vi "GetKey.vi"(10 "node ref in":refnum<data-value>, 11 "RVCLibrary_Bug2 in":refnum<class "RVCLibrary_Bug2.lvclass">) -> (1 "key out":cluster{"(g or v) + h":dbl, "g or v":dbl}, 2 "node ref out":refnum<data-value>, 3 "RVCLibrary_Bug2 out":refnum<class "RVCLibrary_Bug2.lvclass">)   [LabVIEW 2013, in "RVCLibrary_Bug2.lvclass"]
uses:
  RVCLibrary_Bug2.lvclass
  <vilib>/robotics/Navigation/shared/MapNode/AbstractDstarNode/NI_Robotics_AbstractDstarNode.lvclass
  RVCLibrary_Bug2.lvclass/RVCLibrary_Bug2.ctl
panel:
  in  "epsilon current":dbl
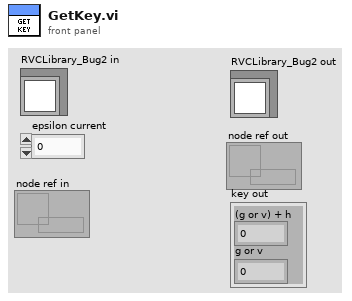
[diagram p1: front panel]
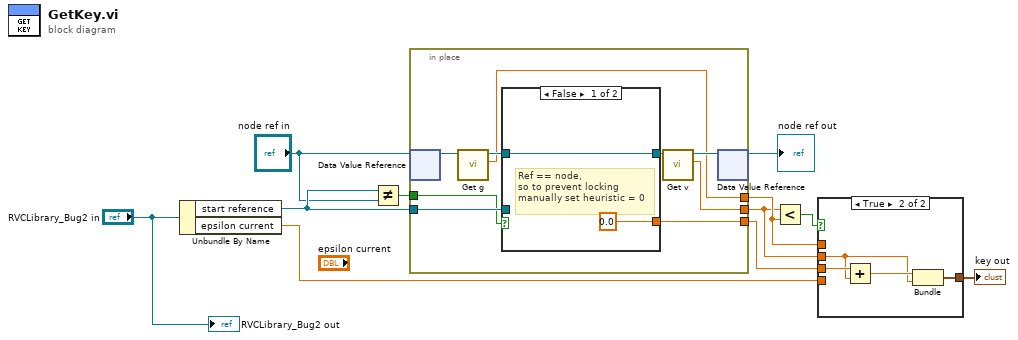
[diagram p0: block diagram]
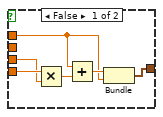
[diagram p2: hidden frame]
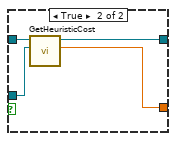
[diagram p3: hidden frame]
diagram:
  n1 = Unbundle By Name("RVCLibrary_Bug2 in") -> ("start reference"=w3:refnum<data-value>, "epsilon current"=w5:dbl)
  n2 = Not Equal?(x=w3, y="node ref in") -> (x != y?=w4:bool)
  n3 = in-place {
    in-place-border: w3 -> [w16]
    in-place-border: [w15] -> w7
    in-place-border: [w14] -> w10
    in-place-border: [w13] -> w8
    in-place-border: w4 -> [w12]
    n4 = in-place-dvr #1("node ref in") -> (w19:refnum<class "NI_Robotics_AbstractDstarNode.lvclass">)  [unwired: 1 out]
    n5 = call <vilib>:"Get g.vi"("AbstractDstarNode in"=w19) -> ("g"=w13:dbl, "AbstractDstarNode out"=w18:refnum<class "NI_Robotics_AbstractDstarNode.lvclass">)  [unwired: 9 in]
    n6 = case shown="False" w12 {
      tunnel: [0.0 ("Hueristic Cost") w26] -> w14
      tunnel: w18 -> [w22 w25]
      tunnel: [w22 w24] -> w17
      tunnel: w16 -> [_ w23]
      frame False {
        # "Ref == node,\nso to prevent locking\nmanually set heuristic = 0"
      }
      frame True {
        n7 = call-dynamic "GetHeuristicCost.vi"("Goal NodeReference"=w23, "AbstractAstarNode in"=w25) -> ("hueristic cost"=w26:dbl, "AbstractAstarNode out"=w24:refnum<class "NI_Robotics_AbstractDstarNode.lvclass">)  [unwired: 7 in, 1 out]
      }
    }
    n8 = call <vilib>:"Get v.vi"("AbstractDstarNode in"=w17) -> ("v"=w15:dbl, "AbstractDstarNode out"=w20:refnum<class "NI_Robotics_AbstractDstarNode.lvclass">)  [unwired: 9 in]
    n9 = in-place-dvr #1(w20) -> (→"node ref out":refnum<data-value>)  [unwired: 1 out]
  }
  n10 = Less?(x=w7, y=w8) -> (x < y?=w6:bool)
  n11 = case shown="True" w6 {
    tunnel: [w27 w36] -> w9
    tunnel: w10 -> [w28 w34]
    tunnel: w7 -> [_ w33]
    tunnel: w8 -> [w30 _]
    tunnel: w5 -> [w29 _]
    frame False {
      n12 = Multiply(x=w29, y=w28) -> (x*y=w31:dbl)
      n13 = Add(x=w30, y=w31) -> (x+y=w32:dbl)
      n14 = Bundle(w32, "g"=w30) -> (w27:cluster{dbl, "g":dbl})  [unwired: 1 in]
    }
    frame True {
      n15 = Add(x=w34, y=w33) -> (x+y=w35:dbl)
      n16 = Bundle(w35, "v"=w33) -> (w36:cluster{dbl, "v":dbl})  [unwired: 1 in]
    }
  }
  "key out" <- w9
  "RVCLibrary_Bug2 out" <- "RVCLibrary_Bug2 in"
